vi "Simulator.vi"() -> ()   [LabVIEW 2013]
panel:
  in  "constants":dbl[](array[numeric])
  out "Front Right":dbl(slide) scale=0.0..1.0
  out "Rear Right":dbl(slide) scale=0.0..1.0
  out "Rear Left":dbl(slide) scale=0.0..1.0
  out "Front Left":dbl(slide) scale=0.0..1.0
  in  "z":dbl
  in  "y":dbl
  in  "x":dbl
  out "Rear Right":dbl(knob) scale=-3.14..3.14
  out "Rear Left":dbl(knob) scale=-3.14..3.14
  out "Front Right":dbl(knob) scale=-3.14..3.14
  out "Front Left":dbl(knob) scale=-3.14..3.14
  in  "Robot Orientation":dbl(knob) scale=-3.14..3.14
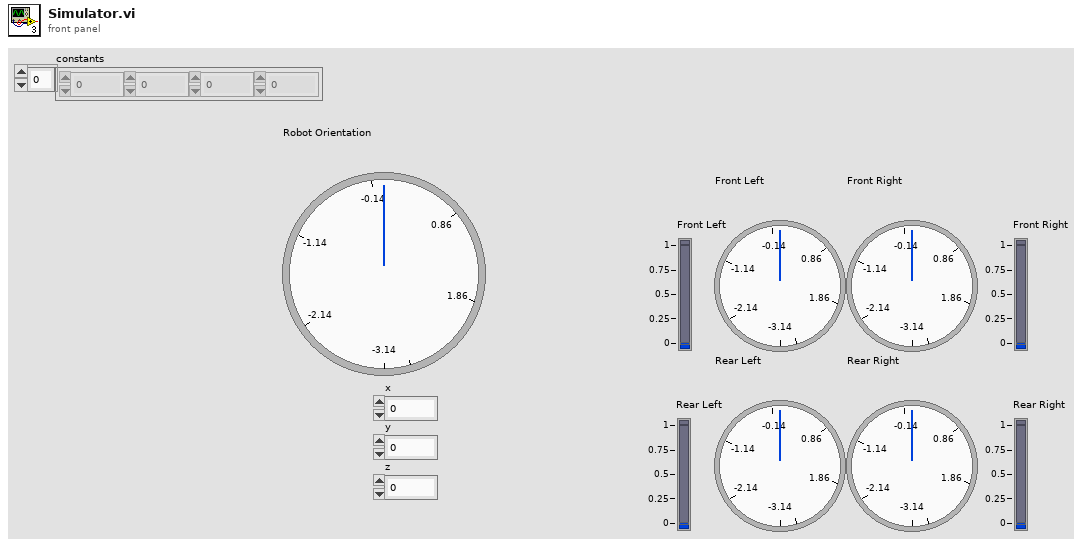
[diagram p1: front panel]
types:
  T1 = enum16{"FrontRight", "FrontLeft", "RearRight", "RearLeft", ""}
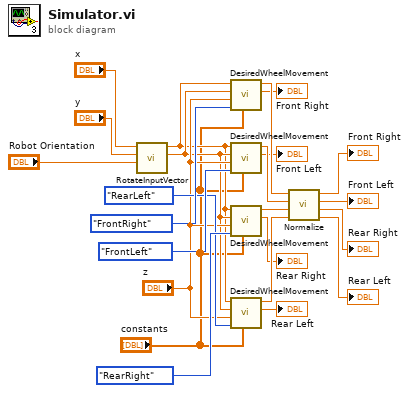
[diagram p0: block diagram]
diagram:
  n1 = call "RotateInputVector.vi"("gyro offset"="Robot Orientation", "y"="y", "x"="x") -> ("y"=w12:dbl, "x"=w11:dbl)  [unwired: 7 in]
  n2 = call "DesiredWheelMovement.vi"("constants"="constants", "wheel"=T1."FrontRight", "z"="z", "y"=w12, "x"=w11) -> ("desired angle (radians)"=→"Front Right":dbl, "desired speed"=w23:dbl)  [unwired: 5 in]
  n3 = call "DesiredWheelMovement.vi"("constants"="constants", "wheel"=T1."FrontLeft", "z"="z", "y"=w12, "x"=w11) -> ("desired angle (radians)"=→"Front Left":dbl, "desired speed"=w22:dbl)  [unwired: 5 in]
  n4 = call "DesiredWheelMovement.vi"("constants"="constants", "wheel"=T1."RearRight", "z"="z", "y"=w12, "x"=w11) -> ("desired angle (radians)"=→"Rear Right":dbl, "desired speed"=w21:dbl)  [unwired: 5 in]
  n5 = call "DesiredWheelMovement.vi"("constants"="constants", "wheel"=T1."RearLeft", "z"="z", "y"=w12, "x"=w11) -> ("desired angle (radians)"=→"Rear Left":dbl, "desired speed"=w20:dbl)  [unwired: 5 in]
  n6 = call "Normalize.vi"("element 4"=w20, "element 3"=w21, "element 2"=w22, "element 1"=w23) -> ("element 4"=→"Rear Left":dbl, "element 3"=→"Rear Right":dbl, "element 2"=→"Front Left":dbl, "element 1"=→"Front Right":dbl)  [unwired: 4 in]
